vi "KillNamedVI.vi"() -> ()   [LabVIEW 2021]
panel:
  out "error out":errorcluster
  in  "VI name to kill":string
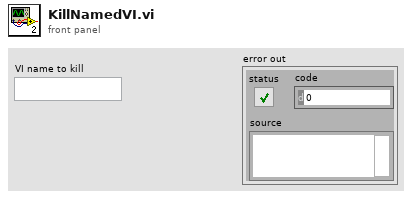
[diagram p1: front panel]
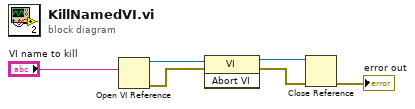
[diagram p0: block diagram]
diagram:
  n1 = Open VI Reference(vi path="VI name to kill") -> (vi reference=w5:refnum<vi>, error out=w4:errorcluster)  [unwired: 5 in]
  n2 = invoke class="VI" method="Abort VI"(reference=w5, error in=w4) -> (reference out=w3:refnum<vi>, error out=w2:errorcluster)  [unwired: 1 in, 1 out]
  n3 = Close Reference(reference=w3, error in (no error)=w2) -> (error out=→"error out":errorcluster)
